vi "system7_60psi.vi"(0 "Presure Regulator AO1":dbl, 1 "Presure Regulator AO2":dbl, 2 "Presure Regulator AO3":dbl, 3 "Presure Regulator AO4":dbl, 4 "Presure Regulator AO5":dbl, 5 "Presure Regulator AO6":dbl, 6 "Presure Regulator AO0":dbl, 7 "Presure Regulator AO 13":dbl, 9 "Presure Regulator AO 14":dbl, 11 "Presure Regulator AO 15":dbl, 14 "Presure Regulator AO7":dbl, 15 "Presure Regulator AO8":dbl, 16 "Presure Regulator AO9":dbl, 17 "Presure Regulator AO10":dbl, 18 "Presure Regulator AO 11":dbl, 19 "Presure Regulator AO 12":dbl) -> ()   [LabVIEW 2015]
uses:
  <vilib>/Tufts CEEO ROS for LabVIEW Software/ROS/MessageBuilding/std_msgs/subs/boolScalar.vi
  <vilib>/express/express shared/transition.llb/Dynamic To Waveform Array.vi
  <vilib>/express/express arith-compare/Formula/Block/exnFormulaBlock how many pts in the wave.vi
  <vilib>/express/express shared/ex_Modify Signal Name.vi
  <vilib>/express/express shared/transition.llb/Waveform Array To Dynamic.vi
  <vilib>/express/express arith-compare/Formula/XNode/ExpressFormulaBlockNode.xnode
panel:
  out "Cluster":cluster{"x":dbl, "y":dbl, "z":dbl}
  in  "reply":bool
  out "Request":string
  in  "DO4":bool
  in  "DO31":bool
  in  "DO30":bool
  in  "DO29":bool
  in  "DO28":bool
  in  "DO27":bool
  in  "DO26":bool
  in  "DO25":bool
  in  "DO24":bool
  in  "DO23":bool
  in  "DO22":bool
  in  "DO21":bool
  in  "DO20":bool
  in  "DO19":bool
  in  "DO18":bool
  in  "DO17":bool
  in  "DO16":bool
  in  "DO15":bool
  in  "DO14":bool
  in  "DO13":bool
  in  "DO12":bool
  in  "DO11":bool
  in  "DO10":bool
  in  "DO9":bool
  in  "DO8":bool
  in  "DO7":bool
  in  "DO6":bool
  in  "DO5":bool
  in  "DO3":bool
  in  "DO2":bool
  in  "DO0":bool
  in  "DO1":bool
  out "Pressure Sensor AI 15":dbl
  out "Pressure Sensor AI 14":dbl
  out "Pressure Sensor AI 13":dbl
  out "Pressure Sensor AI 12":dbl
  out "Pressure Sensor AI 11":dbl
  out "Pressure Sensor AI 10":dbl
  out "Pressure Sensor AI 9":dbl
  out "Pressure Sensor AI 8":dbl
  out "Pressure Sensor AI 7":dbl
  out "Pressure Sensor AI 6":dbl
  out "Pressure Sensor AI 5":dbl
  out "Pressure Sensor AI 4":dbl
  out "Pressure Sensor AI 3":dbl
  out "Pressure Sensor AI 2":dbl
  out "Pressure Sensor AI 1":dbl
  out "Pressure Sensor AI 0":dbl
  out "AI15 Voltage":dbl
  out "AI14 Voltage":dbl
  out "AI13 Voltage":dbl
  out "AI12 Voltage":dbl
  out "AI11 Voltage":dbl
  out "AI10 Voltage":dbl
  out "AI9 Voltage":dbl
  out "AI8 01":dbl
  out "AI7 Voltage":dbl
  out "AI6 Voltage":dbl
  out "AI5 Voltage":dbl
  out "AI4 Voltage":dbl
  out "AI3 Voltage":dbl
  out "AI2 Voltage":dbl
  out "AI0 Voltage":dbl
  out "AI1 Voltage":dbl
  out "error out":errorcluster
  # "ON/Off buttons for valves"
  # "Pressure Desired (PSI)"
  # "Pressure Sensor Readings (PSI)"
  # "Voltage Input From Pressure Sensors (V)"
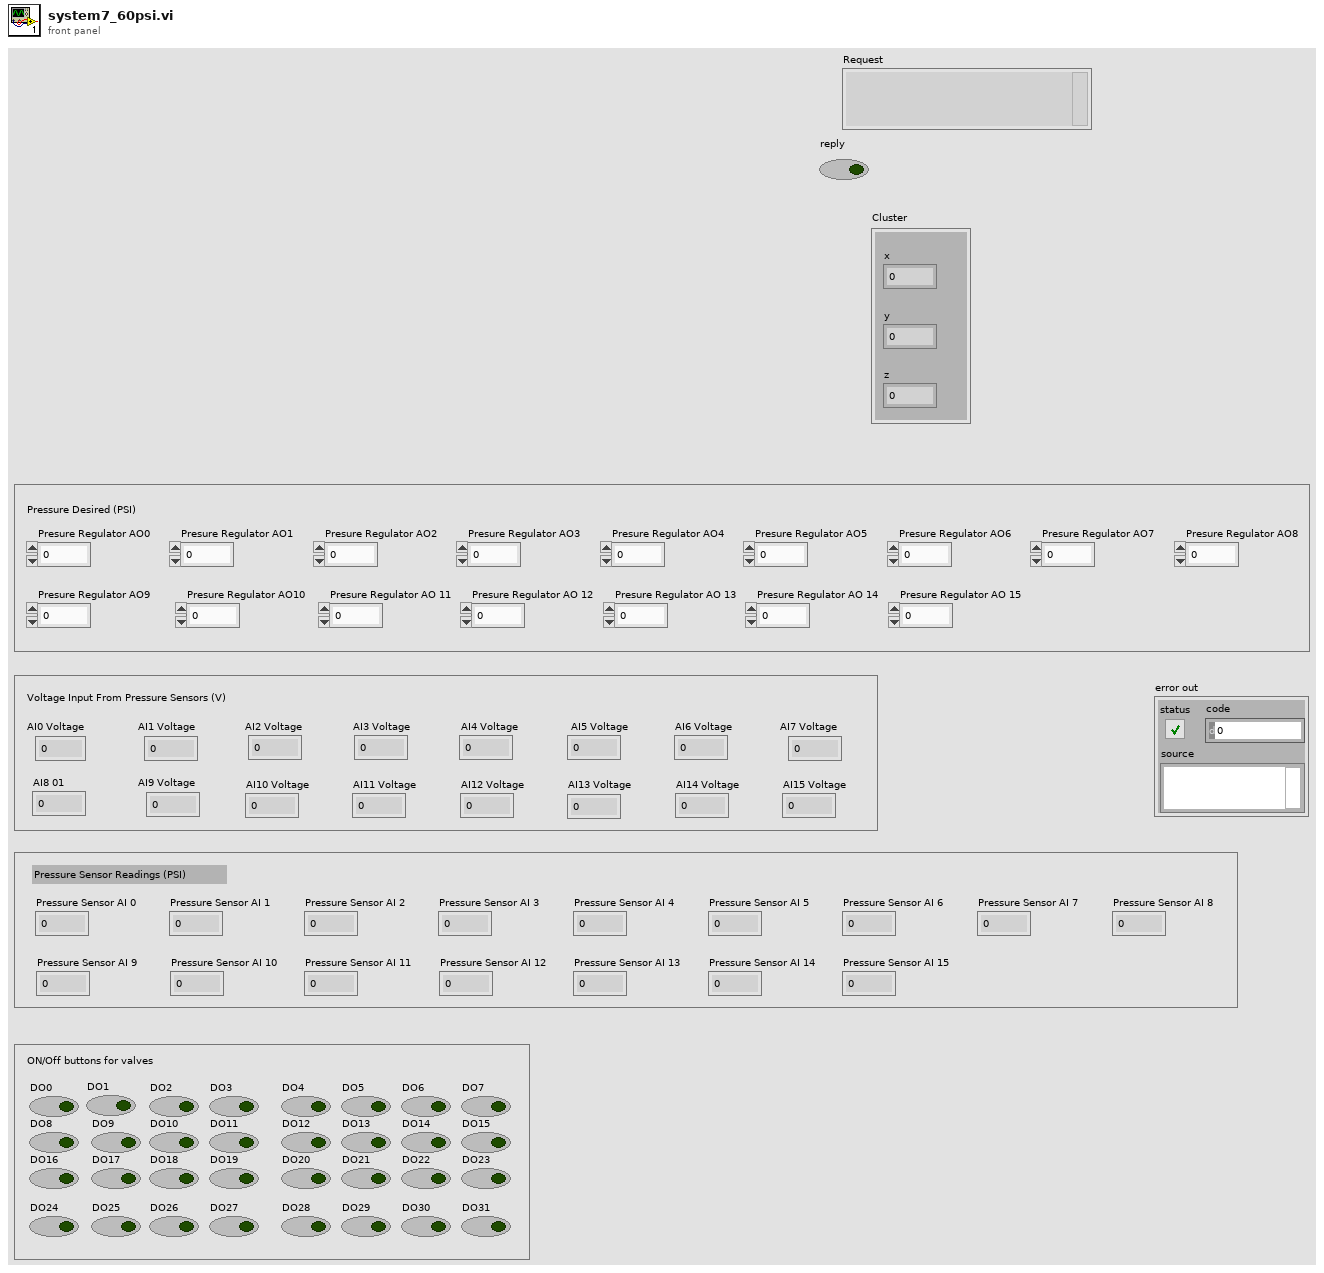
[diagram p1: front panel]
types:
  T1 = typedef "_ROSControl.ctl" = cluster{"topic port":u16, "Node":string, "topic":string, "type":string, "node port":u16, "error ":errorcluster, "Direction":T2, "Update (ms)":u16, "FIFO size":u16}
  T2 = typedef "_ROSDirection.ctl" = enum16{"Node", "Publisher", "Subscriber", "ServiceClient", "ServiceProvider"}
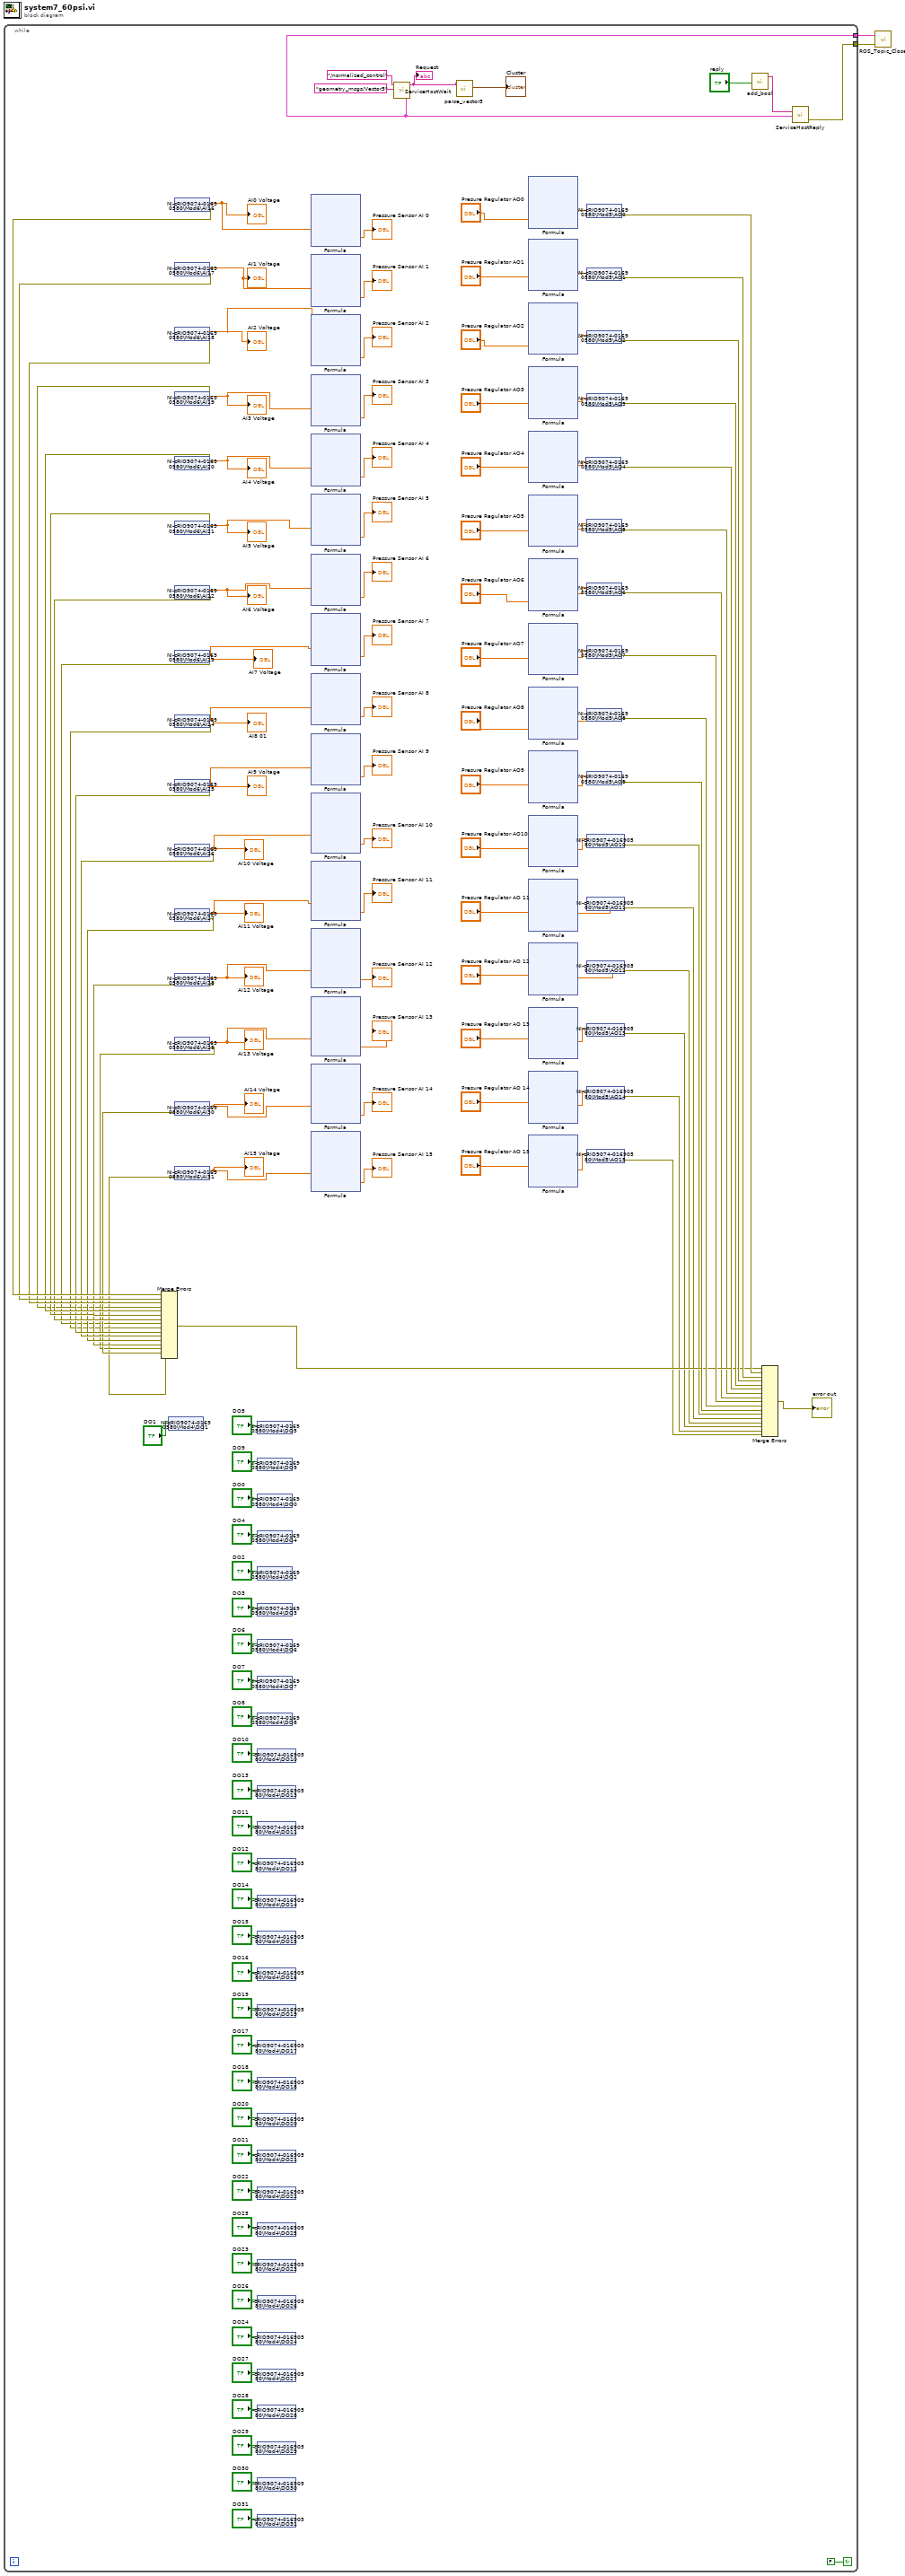
[diagram p0: block diagram]
diagram:
  n1 = while {
    tunnel: [w6] -> w2
    tunnel: [w5] -> w1
    stop <- FALSE continue-if-true
    n2 = shared-variable "NI-cRIO9074-01690580\\Mod4\\DO1"("DO1") -> ()  [unwired: 1 in, 1 out]
    n3 = shared-variable "NI-cRIO9074-01690580\\Mod6\\AI16"() -> (w120:dbl, error out=w132:errorcluster)  [unwired: 1 in]
    "AI0 Voltage" <- w120
    n4 = shared-variable "NI-cRIO9074-01690580\\Mod6\\AI17"() -> (w116:dbl, error out=w131:errorcluster)  [unwired: 1 in]
    "AI1 Voltage" <- w116
    n5 = shared-variable "NI-cRIO9074-01690580\\Mod6\\AI18"() -> (w48:dbl, error out=w130:errorcluster)  [unwired: 1 in]
    "AI2 Voltage" <- w48
    n6 = shared-variable "NI-cRIO9074-01690580\\Mod6\\AI19"() -> (w111:dbl, error out=w47:errorcluster)  [unwired: 1 in]
    "AI3 Voltage" <- w111
    n7 = shared-variable "NI-cRIO9074-01690580\\Mod6\\AI20"() -> (w113:dbl, error out=w129:errorcluster)  [unwired: 1 in]
    "AI4 Voltage" <- w113
    n8 = shared-variable "NI-cRIO9074-01690580\\Mod6\\AI21"() -> (w107:dbl, error out=w128:errorcluster)  [unwired: 1 in]
    "AI5 Voltage" <- w107
    n9 = shared-variable "NI-cRIO9074-01690580\\Mod6\\AI22"() -> (w109:dbl, error out=w127:errorcluster)  [unwired: 1 in]
    "AI6 Voltage" <- w109
    n10 = shared-variable "NI-cRIO9074-01690580\\Mod6\\AI23"() -> (w105:dbl, error out=w45:errorcluster)  [unwired: 1 in]
    "AI7 Voltage" <- w105
    n11 = shared-variable "NI-cRIO9074-01690580\\Mod6\\AI24"() -> (w103:dbl, error out=w44:errorcluster)  [unwired: 1 in]
    "AI8 01" <- w103
    n12 = shared-variable "NI-cRIO9074-01690580\\Mod6\\AI25"() -> (w101:dbl, error out=w126:errorcluster)  [unwired: 1 in]
    "AI9 Voltage" <- w101
    n13 = shared-variable "NI-cRIO9074-01690580\\Mod6\\AI26"() -> (w99:dbl, error out=w125:errorcluster)  [unwired: 1 in]
    "AI10 Voltage" <- w99
    n14 = shared-variable "NI-cRIO9074-01690580\\Mod6\\AI27"() -> (w97:dbl, error out=w124:errorcluster)  [unwired: 1 in]
    "AI11 Voltage" <- w97
    n15 = shared-variable "NI-cRIO9074-01690580\\Mod6\\AI28"() -> (w95:dbl, error out=w123:errorcluster)  [unwired: 1 in]
    "AI12 Voltage" <- w95
    n16 = shared-variable "NI-cRIO9074-01690580\\Mod6\\AI29"() -> (w93:dbl, error out=w46:errorcluster)  [unwired: 1 in]
    "AI13 Voltage" <- w93
    n17 = shared-variable "NI-cRIO9074-01690580\\Mod6\\AI30"() -> (w70:dbl, error out=w71:errorcluster)  [unwired: 1 in]
    "AI14 Voltage" <- w70
    n18 = shared-variable "NI-cRIO9074-01690580\\Mod6\\AI31"() -> (w68:dbl, error out=w12:errorcluster)  [unwired: 1 in]
    "AI15 Voltage" <- w68
    n19 = Merge Errors(w132, w131, w130, w47, w129, w128, w127, w45, w44, w126, w125, w124, w123, w46, w71, w12) -> (w122:errorcluster)
    n20 = shared-variable "NI-cRIO9074-01690580\\Mod4\\DO5"("DO5") -> ()  [unwired: 1 in, 1 out]
    n21 = shared-variable "NI-cRIO9074-01690580\\Mod4\\DO9"("DO9") -> ()  [unwired: 1 in, 1 out]
    n22 = shared-variable "NI-cRIO9074-01690580\\Mod4\\DO0"("DO0") -> ()  [unwired: 1 in, 1 out]
    n23 = shared-variable "NI-cRIO9074-01690580\\Mod4\\DO4"("DO4") -> ()  [unwired: 1 in, 1 out]
    n24 = shared-variable "NI-cRIO9074-01690580\\Mod4\\DO2"("DO2") -> ()  [unwired: 1 in, 1 out]
    n25 = shared-variable "NI-cRIO9074-01690580\\Mod4\\DO3"("DO3") -> ()  [unwired: 1 in, 1 out]
    n26 = shared-variable "NI-cRIO9074-01690580\\Mod4\\DO6"("DO6") -> ()  [unwired: 1 in, 1 out]
    n27 = shared-variable "NI-cRIO9074-01690580\\Mod4\\DO7"("DO7") -> ()  [unwired: 1 in, 1 out]
    n28 = shared-variable "NI-cRIO9074-01690580\\Mod4\\DO8"("DO8") -> ()  [unwired: 1 in, 1 out]
    n29 = shared-variable "NI-cRIO9074-01690580\\Mod4\\DO10"("DO10") -> ()  [unwired: 1 in, 1 out]
    n30 = shared-variable "NI-cRIO9074-01690580\\Mod4\\DO13"("DO13") -> ()  [unwired: 1 in, 1 out]
    n31 = shared-variable "NI-cRIO9074-01690580\\Mod4\\DO11"("DO11") -> ()  [unwired: 1 in, 1 out]
    n32 = shared-variable "NI-cRIO9074-01690580\\Mod4\\DO12"("DO12") -> ()  [unwired: 1 in, 1 out]
    n33 = shared-variable "NI-cRIO9074-01690580\\Mod4\\DO14"("DO14") -> ()  [unwired: 1 in, 1 out]
    n34 = shared-variable "NI-cRIO9074-01690580\\Mod4\\DO15"("DO15") -> ()  [unwired: 1 in, 1 out]
    n35 = shared-variable "NI-cRIO9074-01690580\\Mod4\\DO16"("DO16") -> ()  [unwired: 1 in, 1 out]
    n36 = shared-variable "NI-cRIO9074-01690580\\Mod4\\DO19"("DO19") -> ()  [unwired: 1 in, 1 out]
    n37 = shared-variable "NI-cRIO9074-01690580\\Mod4\\DO17"("DO17") -> ()  [unwired: 1 in, 1 out]
    n38 = shared-variable "NI-cRIO9074-01690580\\Mod4\\DO18"("DO18") -> ()  [unwired: 1 in, 1 out]
    n39 = shared-variable "NI-cRIO9074-01690580\\Mod4\\DO20"("DO20") -> ()  [unwired: 1 in, 1 out]
    n40 = shared-variable "NI-cRIO9074-01690580\\Mod4\\DO21"("DO21") -> ()  [unwired: 1 in, 1 out]
    n41 = shared-variable "NI-cRIO9074-01690580\\Mod4\\DO22"("DO22") -> ()  [unwired: 1 in, 1 out]
    n42 = shared-variable "NI-cRIO9074-01690580\\Mod4\\DO25"("DO25") -> ()  [unwired: 1 in, 1 out]
    n43 = shared-variable "NI-cRIO9074-01690580\\Mod4\\DO23"("DO23") -> ()  [unwired: 1 in, 1 out]
    n44 = shared-variable "NI-cRIO9074-01690580\\Mod4\\DO26"("DO26") -> ()  [unwired: 1 in, 1 out]
    n45 = shared-variable "NI-cRIO9074-01690580\\Mod4\\DO24"("DO24") -> ()  [unwired: 1 in, 1 out]
    n46 = shared-variable "NI-cRIO9074-01690580\\Mod4\\DO27"("DO27") -> ()  [unwired: 1 in, 1 out]
    n47 = shared-variable "NI-cRIO9074-01690580\\Mod4\\DO28"("DO28") -> ()  [unwired: 1 in, 1 out]
    n48 = shared-variable "NI-cRIO9074-01690580\\Mod4\\DO29"("DO29") -> ()  [unwired: 1 in, 1 out]
    n49 = shared-variable "NI-cRIO9074-01690580\\Mod4\\DO30"("DO30") -> ()  [unwired: 1 in, 1 out]
    n50 = shared-variable "NI-cRIO9074-01690580\\Mod4\\DO31"("DO31") -> ()  [unwired: 1 in, 1 out]
    n51 = xnode "Formula"("X1"=w120) -> ("Result"=→"Pressure Sensor AI 0":dbl)  [unwired: 1 in, 1 out]
    n52 = xnode "Formula"("X1"=w116) -> ("Result"=→"Pressure Sensor AI 1":dbl)  [unwired: 1 in, 1 out]
    n53 = xnode "Formula"("X1"=w48) -> ("Result"=→"Pressure Sensor AI 2":dbl)  [unwired: 1 in, 1 out]
    n54 = xnode "Formula"("X1"=w111) -> ("Result"=→"Pressure Sensor AI 3":dbl)  [unwired: 1 in, 1 out]
    n55 = xnode "Formula"("X1"=w113) -> ("Result"=→"Pressure Sensor AI 4":dbl)  [unwired: 1 in, 1 out]
    n56 = xnode "Formula"("X1"=w107) -> ("Result"=→"Pressure Sensor AI 5":dbl)  [unwired: 1 in, 1 out]
    n57 = xnode "Formula"("X1"=w109) -> ("Result"=→"Pressure Sensor AI 6":dbl)  [unwired: 1 in, 1 out]
    n58 = xnode "Formula"("X1"=w105) -> ("Result"=→"Pressure Sensor AI 7":dbl)  [unwired: 1 in, 1 out]
    n59 = xnode "Formula"("X1"=w103) -> ("Result"=→"Pressure Sensor AI 8":dbl)  [unwired: 1 in, 1 out]
    n60 = xnode "Formula"("X1"=w101) -> ("Result"=→"Pressure Sensor AI 9":dbl)  [unwired: 1 in, 1 out]
    n61 = xnode "Formula"("X1"=w99) -> ("Result"=→"Pressure Sensor AI 10":dbl)  [unwired: 1 in, 1 out]
    n62 = xnode "Formula"("X1"=w97) -> ("Result"=→"Pressure Sensor AI 11":dbl)  [unwired: 1 in, 1 out]
    n63 = xnode "Formula"("X1"=w95) -> ("Result"=→"Pressure Sensor AI 12":dbl)  [unwired: 1 in, 1 out]
    n64 = xnode "Formula"("X1"=w93) -> ("Result"=→"Pressure Sensor AI 13":dbl)  [unwired: 1 in, 1 out]
    n65 = xnode "Formula"("X1"=w70) -> ("Result"=→"Pressure Sensor AI 14":dbl)  [unwired: 1 in, 1 out]
    n66 = xnode "Formula"("X1"=w68) -> ("Result"=→"Pressure Sensor AI 15":dbl)  [unwired: 1 in, 1 out]
    n67 = call <userlib>:"ServiceHostWait.vi"("Topic"="/normalized_control", "Type"="geometry_msgs/Vector3") -> ("Request"=w3:string, "Service ROS info out"=w5:T1)  [unwired: 3 in]
    "Request" <- w3
    n68 = call <vilib>:"parse_vector3.vi"("msg in"=w3) -> ("Vector3"=→"Cluster":cluster{"x":dbl, "y":dbl, "z":dbl})  [unwired: 4 in, 2 out]
    n69 = xnode "Formula"("Pressure"="Presure Regulator AO0") -> ("Result"=w118:dbl)  [unwired: 1 in, 1 out]
    n70 = xnode "Formula"("Pressure"="Presure Regulator AO1") -> ("Result"=w87:dbl)  [unwired: 1 in, 1 out]
    n71 = xnode "Formula"("Pressure"="Presure Regulator AO2") -> ("Result"=w89:dbl)  [unwired: 1 in, 1 out]
    n72 = xnode "Formula"("Pressure"="Presure Regulator AO3") -> ("Result"=w85:dbl)  [unwired: 1 in, 1 out]
    n73 = xnode "Formula"("Pressure"="Presure Regulator AO4") -> ("Result"=w83:dbl)  [unwired: 1 in, 1 out]
    n74 = xnode "Formula"("Pressure"="Presure Regulator AO5") -> ("Result"=w81:dbl)  [unwired: 1 in, 1 out]
    n75 = xnode "Formula"("Pressure"="Presure Regulator AO6") -> ("Result"=w78:dbl)  [unwired: 1 in, 1 out]
    n76 = xnode "Formula"("Pressure"="Presure Regulator AO7") -> ("Result"=w76:dbl)  [unwired: 1 in, 1 out]
    n77 = xnode "Formula"("Pressure"="Presure Regulator AO8") -> ("Result"=w74:dbl)  [unwired: 1 in, 1 out]
    n78 = xnode "Formula"("Pressure"="Presure Regulator AO9") -> ("Result"=w72:dbl)  [unwired: 1 in, 1 out]
    n79 = xnode "Formula"("Pressure"="Presure Regulator AO10") -> ("Result"=w65:dbl)  [unwired: 1 in, 1 out]
    n80 = xnode "Formula"("Pressure"="Presure Regulator AO 11") -> ("Result"=w62:dbl)  [unwired: 1 in, 1 out]
    n81 = xnode "Formula"("Pressure"="Presure Regulator AO 12") -> ("Result"=w59:dbl)  [unwired: 1 in, 1 out]
    n82 = xnode "Formula"("Pressure"="Presure Regulator AO 13") -> ("Result"=w56:dbl)  [unwired: 1 in, 1 out]
    n83 = xnode "Formula"("Pressure"="Presure Regulator AO 14") -> ("Result"=w53:dbl)  [unwired: 1 in, 1 out]
    n84 = xnode "Formula"("Pressure"="Presure Regulator AO 15") -> ("Result"=w50:dbl)  [unwired: 1 in, 1 out]
    n85 = shared-variable "NI-cRIO9074-01690580\\Mod5\\AO4"(w83) -> (error out=w136:errorcluster)  [unwired: 1 in]
    n86 = shared-variable "NI-cRIO9074-01690580\\Mod5\\AO0"(w118) -> (error out=w141:errorcluster)  [unwired: 1 in]
    n87 = shared-variable "NI-cRIO9074-01690580\\Mod5\\AO1"(w87) -> (error out=w139:errorcluster)  [unwired: 1 in]
    n88 = shared-variable "NI-cRIO9074-01690580\\Mod5\\AO2"(w89) -> (error out=w138:errorcluster)  [unwired: 1 in]
    n89 = shared-variable "NI-cRIO9074-01690580\\Mod5\\AO3"(w85) -> (error out=w137:errorcluster)  [unwired: 1 in]
    n90 = shared-variable "NI-cRIO9074-01690580\\Mod5\\AO5"(w81) -> (error out=w91:errorcluster)  [unwired: 1 in]
    n91 = shared-variable "NI-cRIO9074-01690580\\Mod5\\AO6"(w78) -> (error out=w80:errorcluster)  [unwired: 1 in]
    n92 = shared-variable "NI-cRIO9074-01690580\\Mod5\\AO7"(w76) -> (error out=w135:errorcluster)  [unwired: 1 in]
    n93 = shared-variable "NI-cRIO9074-01690580\\Mod5\\AO8"(w74) -> (error out=w134:errorcluster)  [unwired: 1 in]
    n94 = shared-variable "NI-cRIO9074-01690580\\Mod5\\AO9"(w72) -> (error out=w133:errorcluster)  [unwired: 1 in]
    n95 = shared-variable "NI-cRIO9074-01690580\\Mod5\\AO10"(w65) -> (error out=w64:errorcluster)  [unwired: 1 in]
    n96 = shared-variable "NI-cRIO9074-01690580\\Mod5\\AO11"(w62) -> (error out=w61:errorcluster)  [unwired: 1 in]
    n97 = shared-variable "NI-cRIO9074-01690580\\Mod5\\AO12"(w59) -> (error out=w58:errorcluster)  [unwired: 1 in]
    n98 = shared-variable "NI-cRIO9074-01690580\\Mod5\\AO13"(w56) -> (error out=w55:errorcluster)  [unwired: 1 in]
    n99 = shared-variable "NI-cRIO9074-01690580\\Mod5\\AO14"(w53) -> (error out=w52:errorcluster)  [unwired: 1 in]
    n100 = shared-variable "NI-cRIO9074-01690580\\Mod5\\AO15"(w50) -> (error out=w49:errorcluster)  [unwired: 1 in]
    n101 = call-poly <vilib>:"add_bool.vi"("Boolean"="reply") -> ("msg out"=w8:string)  [unwired: 4 in]
    n102 = Merge Errors(w122, w141, w139, w138, w137, w136, w91, w80, w135, w134, w133, w64, w61, w58, w55, w52, w49) -> (→"error out":errorcluster)
    n103 = call <userlib>:"ServiceHostReply.vi"("Service ROS info in"=w5, "Reply"=w8) -> ("error out"=w6:errorcluster)  [unwired: 2 in]
  }
  n104 = call <userlib>:"ROS_Topic_Close.vi"("error in"=w2, "ROS in"=w1) -> ()  [unwired: 2 in, 1 out]
